vi "JSON to LVObject - Descendant - Returns Matching Type.vi"() -> ()   [LabVIEW 2017, in "Tests.lvlib" / "Type Name Handling.lvlib"]
uses:
  Temperature Forecast/Temperature Forecast.lvclass
  Weather Forecast/Weather Forecast.lvclass
  Flatten To JSON Object/Flatten To JSON Object.lvclass
  Flatten To JSON Object/Type Name Handling.ctl
  Flatten To JSON Object/Flatten To JSON Object.lvclass/Flatten To JSON Object.ctl
  Flatten To JSON Object/Write Type Name Handling.vi
  <vilib>/addons/_JKI Toolkits/Caraya/classes/Assert/Assert Equal Value and Type_Variant.vi
  Type Name Handling.lvlib
  <vilib>/addons/_JKI Toolkits/Caraya/classes/Test/Test.lvclass
  <vilib>/addons/_JKI Toolkits/Caraya/classes/Assert/Assert.lvclass
panel:
  out "error out":errorcluster
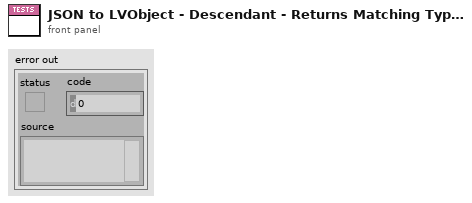
[diagram p1: front panel]
types:
  T1 = typedef "Flatten To JSON Object.lvclass/Type Name Handling.ctl" = enum16{"None", "Inline"}
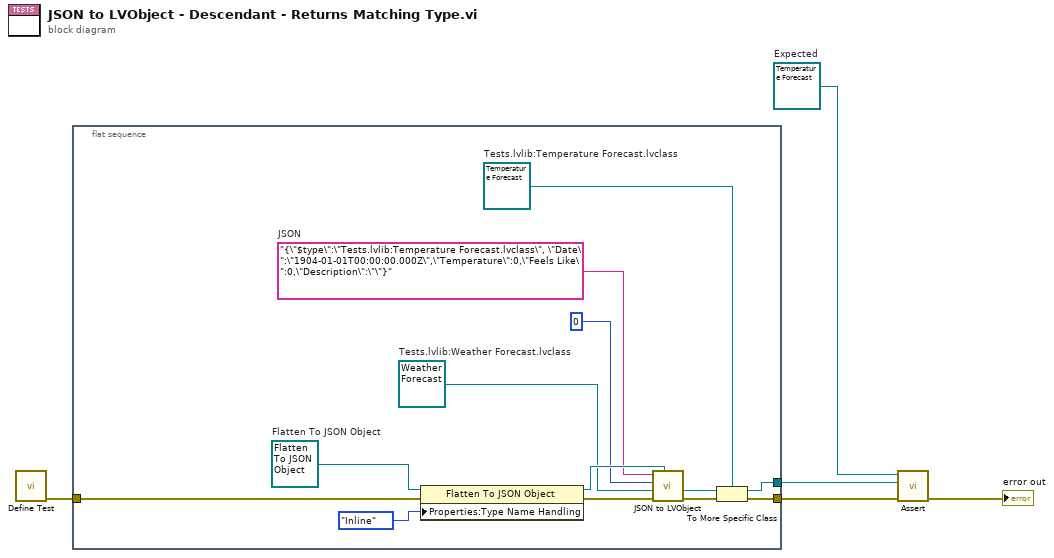
[diagram p0: block diagram]
diagram:
  w1 = refnum<class "Temperature Forecast.lvclass"> refnum  # Expected
  n1 = call <vilib>:"Define Test.vi"() -> ("error out"=w5:errorcluster)  [unwired: 11 in]
  n2 = flat-sequence {
    tunnel: w5 -> [w16]
    tunnel: [w8] -> w4
    tunnel: [w10] -> w3
    frame #0 {
      w6 = refnum<class "Temperature Forecast.lvclass"> refnum  # Tests.lvlib:Temperature Forecast.lvclass
      w13 = "{\"$type\":\"Tests.lvlib:Temperature Forecast.lvclass\", \"Date\":\"1904-01-01T00:00:00.000Z\",\"Temperature\":0,\"Feels Like\":0,\"Description\":\"\"}"  # JSON
      w18 = refnum<class "Flatten To JSON Object.lvclass"> refnum  # Flatten To JSON Object
      w7 = refnum<class "Weather Forecast.lvclass"> refnum  # Tests.lvlib:Weather Forecast.lvclass
      n3 = property class="Flatten To JSON Object"(reference=w18, error in=w16, "Properties:Type Name Handling"=Type_Name_Handling."Inline" ("Type Name Handling")) -> (reference out=w14:refnum<class "Flatten To JSON Object.lvclass">, error out=w15:errorcluster)
      n4 = call-dynamic "JSON to LVObject.vi"("Flatten To JSON Object in"=w14, "error in (no error)"=w15, "Object Type"=w7, "Offset"=0, "JSON"=w13) -> ("error out"=w9:errorcluster, "Object"=w12:refnum<class>)  [unwired: 5 in]
      n5 = To More Specific Class(target class=w6, reference=w12, error in=w9) -> (specific class reference=w10:refnum<class "Temperature Forecast.lvclass">, error out=w8:errorcluster)
    }
  }
  n6 = call-poly <vilib>:"Assert.vi"("error in (no error)"=w4, "Y"=w3, "X"=w1) -> ("error out"=→"error out":errorcluster)  [unwired: 8 in]
